vi "Simple_DAQ_AnalogIO.ProcCases.vi"(0 "i ref in":refnum<vi>, 1 "selector":string, 2 "Data":T1, 3 "call cluster":T2={"Object"="", "Selector"="", "CallType"=enum."synchronous", "Async Object"="", "Async Selector"="", "Data Descriptor"="", "Data"=[], "Error #"=0, "Expire"=0}, 5 "error in (no error)":errorcluster) -> (14 "i ref out":refnum<vi>, 17 "answer cluster":T2={"Object"="", "Selector"="", "CallType"=enum."synchronous", "Async Object"="", "Async Selector"="", "Data Descriptor"="", "Data"=[], "Error #"=0, "Expire"=0}, 19 "error out":errorcluster)   [LabVIEW 2014, in "Simple_DAQ_AnalogIO.lvlib"]
doc: "This method is called by a process from within the default case in the event loop. The methods of a class that are linked to events will be called from THIS method. Add your code here."
uses:
  Simple_DAQ_AnalogIO.lvlib
  CS_Core/CSSystem/CoreDefs/CoreDefs.call_type.ctl
  CS_Core/BaseProcess/BaseProcess.descriptor string definition.ctl
  CS_Core/CSSystem/CoreDefs/CoreDefs.rawDataType.ctl
  CS_Core/CSSystem/CoreLib/CoreLib.string 2 byte array.vi
  CS_Core/CSSystem/CoreLib/CoreLib.double 2 byte array.vi
  CS_Core/CSSystem/CoreLib/CoreLib.byte array 2 double.vi
  CS_Core/CSSystem/CoreLib/CoreLib.byte array 2 int.vi
  CS_Core/CSSystem/CoreLib/CoreLib.lvlib
  CS_Core/BaseProcess/BaseProcess.lvlib
  CS_Core/CSApplicationBaseClasses/PSChannelBase/PSChannelBase.lvlib
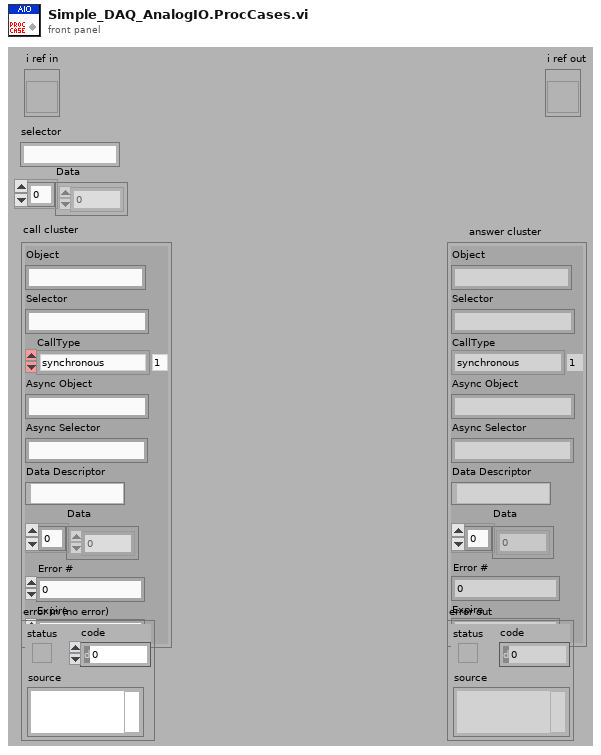
[diagram p1: front panel]
types:
  T1 = typedef "CoreDefs.rawDataType.ctl" = i8[]
  T2 = typedef "CoreDefs.call_type.ctl" = cluster{"Object":string, "Selector":string, "CallType":enum16{"simple", "synchronous", "asynchronous"}, "Async Object":string, "Async Selector":string, "Data Descriptor":T3, "Data":T1, "Error #":i32, "Expire":u32}
  T3 = typedef "BaseProcess.lvlib/BaseProcess.descriptor string definition.ctl" = string
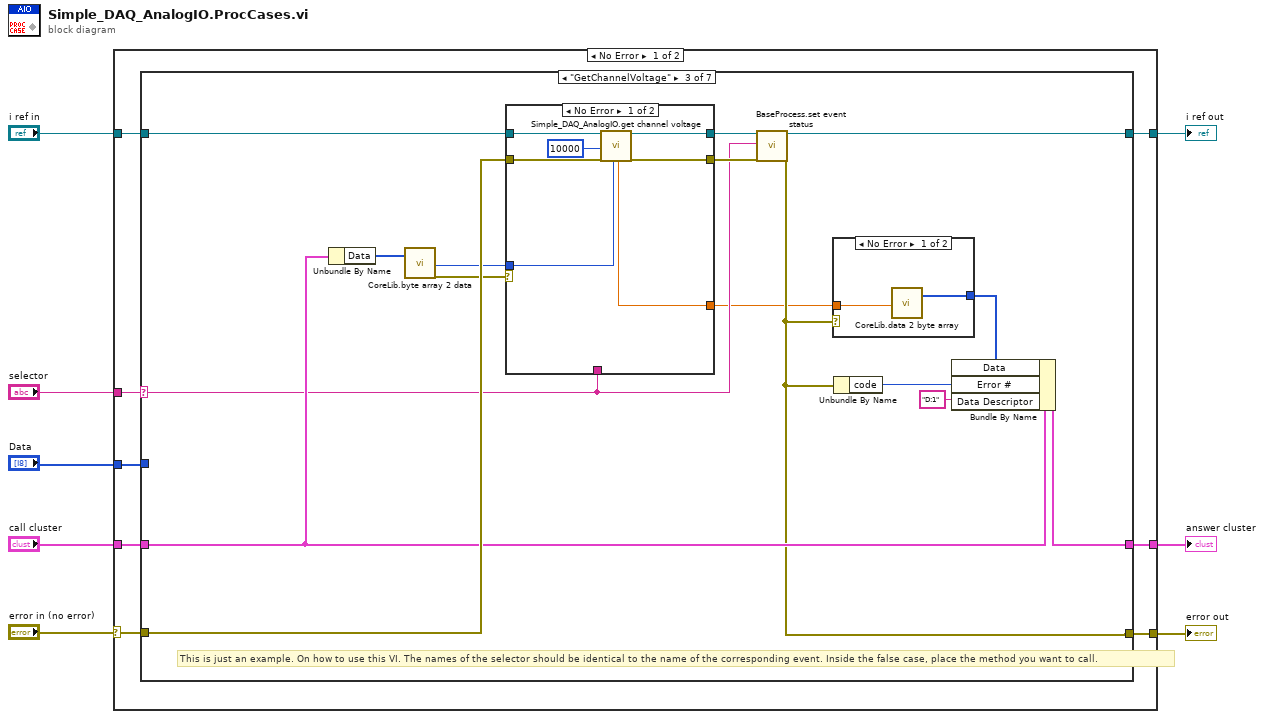
[diagram p0: block diagram]
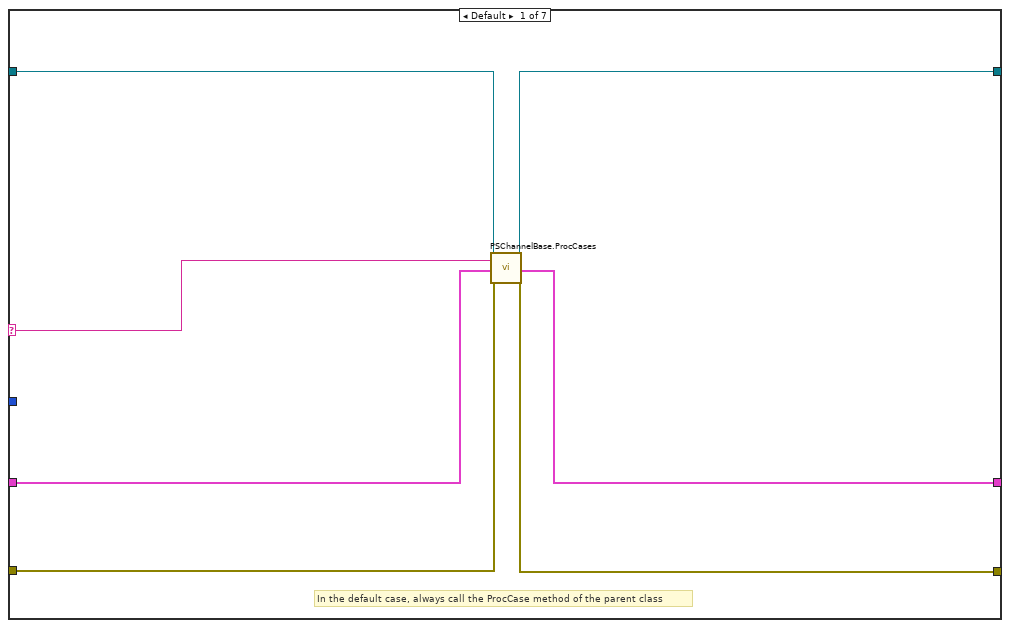
[diagram p2: hidden frame]
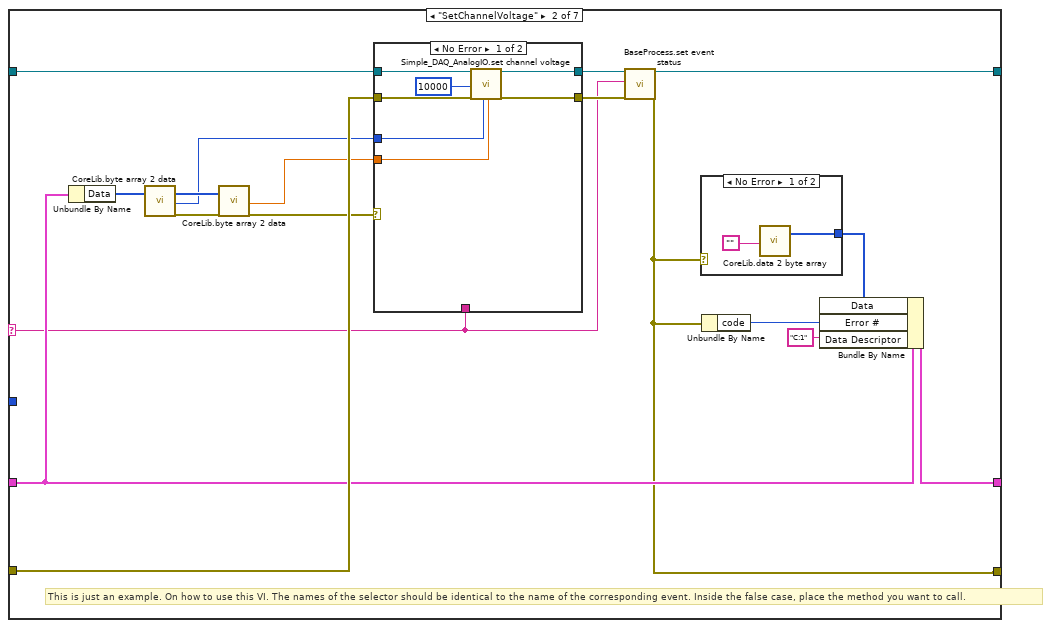
[diagram p3: hidden frame]
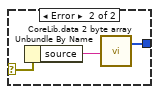
[diagram p4: hidden frame]
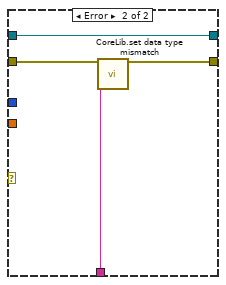
[diagram p5: hidden frame]
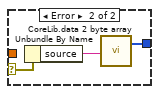
[diagram p6: hidden frame]
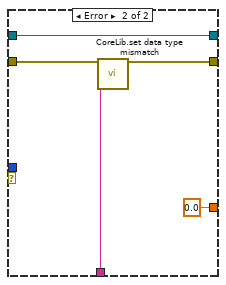
[diagram p7: hidden frame]
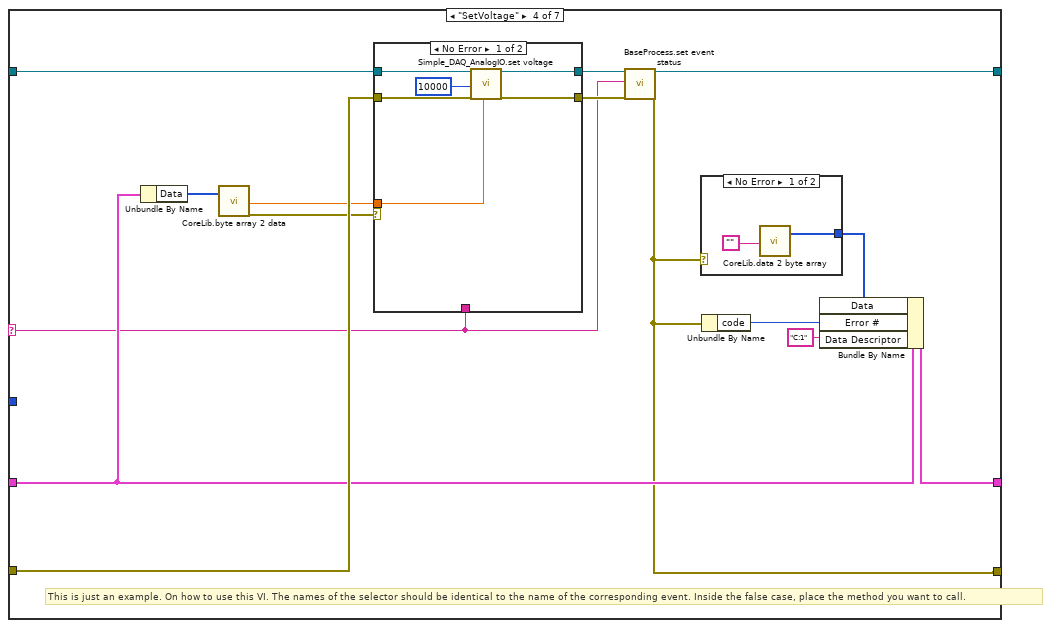
[diagram p8: hidden frame]
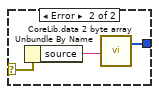
[diagram p9: hidden frame]
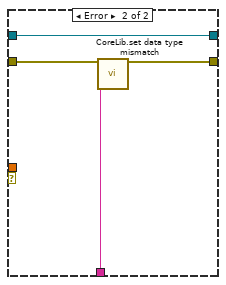
[diagram p10: hidden frame]
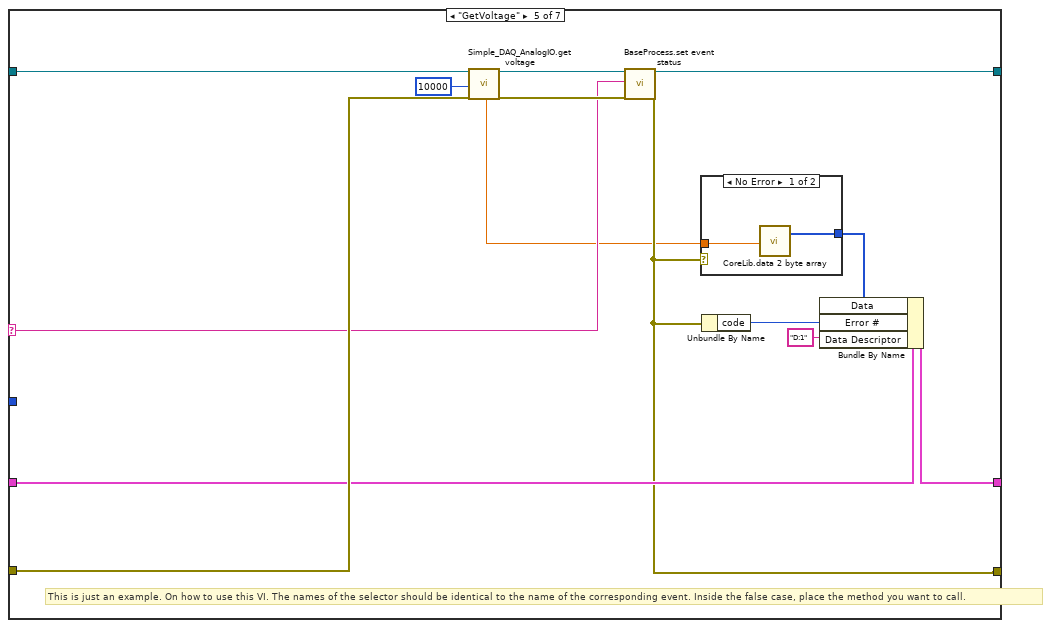
[diagram p11: hidden frame]
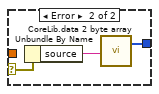
[diagram p12: hidden frame]
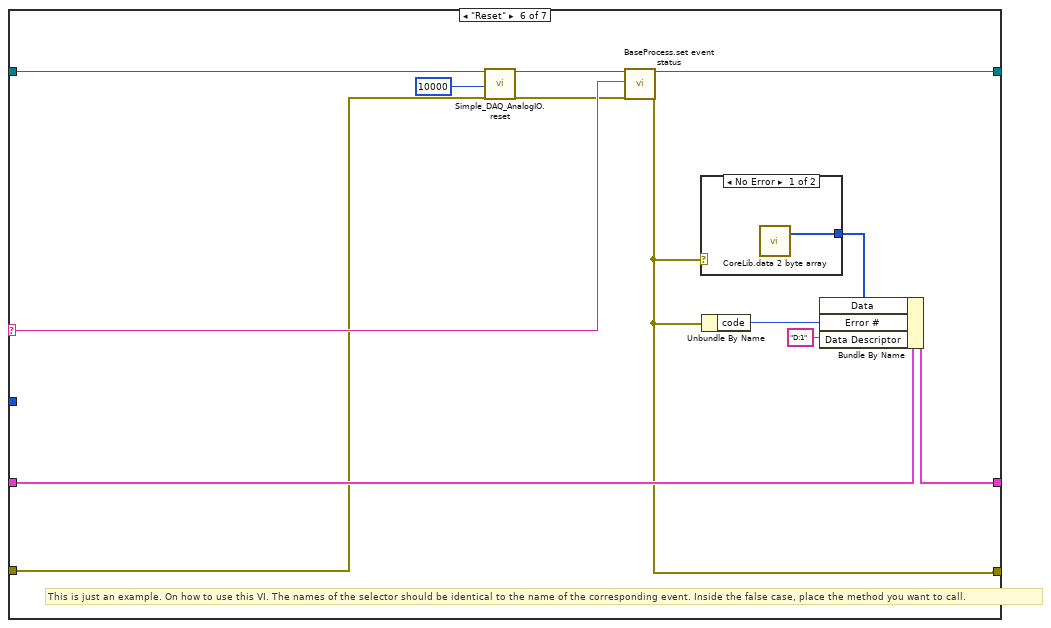
[diagram p13: hidden frame]
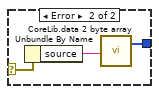
[diagram p14: hidden frame]
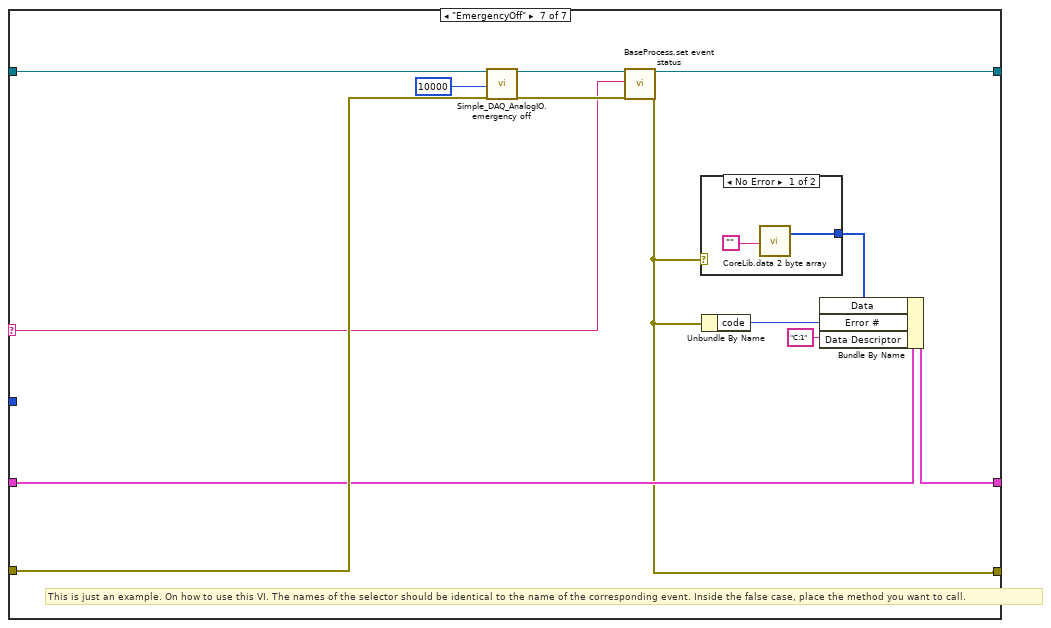
[diagram p15: hidden frame]
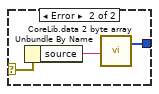
[diagram p16: hidden frame]
diagram:
  n1 = case shown="No Error" "error in (no error)" {
    selector: "error in (no error)" -> [w9 w175]
    tunnel: "selector" -> [w16 _]
    tunnel: [w15 w176] -> w7
    tunnel: "Data" -> [w14 _]
    tunnel: "call cluster" -> [w13 w176]
    tunnel: "i ref in" -> [w12 w177]
    tunnel: [w11 w177] -> w3
    tunnel: [w10 w175] -> w2
    frame No Error {
      n2 = case shown="\"GetChannelVoltage\"" w16 {
        selector: w16 -> [w18 w32 w64 w96 w125 w147 w160]
        tunnel: w14 -> [_ _ _ _ _ _ _]
        tunnel: w12 -> [w17 w41 w73 w105 w134 w144 w169]
        tunnel: [w23 w31 w63 w95 w124 w146 w159] -> w11
        tunnel: w13 -> [w19 w38 w70 w102 w131 w151 w166]
        tunnel: [w20 w37 w69 w101 w130 w150 w165] -> w15
        tunnel: w9 -> [w22 w40 w72 w104 w133 w141 w168]
        tunnel: [w21 w33 w65 w97 w126 w148 w161] -> w10
        frame Default {
          # "In the default case, always call the ProcCase method of the parent class"
          n3 = call "PSChannelBase.ProcCases.vi"("i ref in"=w17, "selector"=w18, "call cluster"=w19, "error in (no error)"=w22) -> ("i ref out"=w23:refnum<vi>, "answer cluster"=w20:T2, "error out"=w21:errorcluster)  [unwired: 13 in]
        }
        frame "SetChannelVoltage" {
          # "This is just an example. On how to use this VI. The names of the selector should be identical to the name of the corresponding event. Inside the false case, place the method you want to call."
          n4 = Unbundle By Name(w38) -> ("Data"=w29:T1)
          n5 = call-poly "CoreLib.byte array 2 data.vi"("byteArray"=w29) -> ("byteArray out"=w27:T1, "i32"=w25:i32, "error out"=w28:errorcluster)  [unwired: 16 in]
          n6 = call-poly "CoreLib.byte array 2 data.vi"("byteArray"=w27, "error in (no error)"=w28) -> ("d64"=w24:dbl, "error out"=w26:errorcluster)  [unwired: 15 in, 1 out]
          n7 = case shown="No Error" w26 {
            tunnel: [w51 w57] -> w35
            tunnel: w41 -> [w52 w57]
            tunnel: w40 -> [w53 w56]
            tunnel: [w50 w55] -> w34
            tunnel: w24 -> [w47 _]
            tunnel: w32 -> [_ w54]
            tunnel: w25 -> [w48 _]
            frame No Error {
              n8 = call "Simple_DAQ_AnalogIO.set channel voltage.vi"("i ref in"=w52, "Timeout"=10000, "error in"=w53, "channel_index"=w48, "voltage"=w47) -> ("i ref out"=w51:refnum<vi>, "error out"=w50:errorcluster)  [unwired: 12 in, 1 out]
            }
            frame Error {
              n9 = call "CoreLib.set data type mismatch.vi"("error in (no error)"=w56, "error source"=w54) -> ("error out"=w55:errorcluster)  [unwired: 17 in]
            }
          }
          n10 = call "BaseProcess.set event status.vi"("i ref in"=w35, "EventStatus"=w32, "error in (no error)"=w34) -> ("i ref out"=w31:refnum<vi>, "error out"=w33:errorcluster)  [unwired: 14 in, 1 out]
          n11 = case shown="No Error" w33 {
            selector: w33 -> [_ w46]
            tunnel: [w43 w45] -> w36
            frame No Error {
              n12 = call-poly "CoreLib.data 2 byte array.vi"("string"="") -> ("byteArray out"=w43:T1)  [unwired: 18 in]
            }
            frame Error {
              n13 = Unbundle By Name(w46) -> ("source"=w44:string)
              n14 = call-poly "CoreLib.data 2 byte array.vi"("string"=w44) -> ("byteArray out"=w45:T1)  [unwired: 18 in]
            }
          }
          n15 = Unbundle By Name(w33) -> ("code"=w39:i32)
          n16 = Bundle By Name(cluster=w38, "Data"=w36, "Error #"=w39, "Data Descriptor"="C:1") -> (w37:T2)
        }
        frame "GetChannelVoltage" {
          # "This is just an example. On how to use this VI. The names of the selector should be identical to the name of the corresponding event. Inside the false case, place the method you want to call."
          n17 = Unbundle By Name(w70) -> ("Data"=w61:T1)
          n18 = call-poly "CoreLib.byte array 2 data.vi"("byteArray"=w61) -> ("i32"=w60:i32, "error out"=w59:errorcluster)  [unwired: 16 in, 1 out]
          n19 = case shown="No Error" w59 {
            tunnel: [w83 w90] -> w67
            tunnel: w73 -> [w84 w90]
            tunnel: w72 -> [w85 w89]
            tunnel: [w82 w88] -> w66
            tunnel: w64 -> [_ w87]
            tunnel: w60 -> [w80 _]
            tunnel: [w79 0.0 ("voltage")] -> w58
            frame No Error {
              n20 = call "Simple_DAQ_AnalogIO.get channel voltage.vi"("i ref in"=w84, "Timeout"=10000, "error in"=w85, "channel_index"=w80) -> ("voltage"=w79:dbl, "i ref out"=w83:refnum<vi>, "error out"=w82:errorcluster)  [unwired: 12 in, 1 out]
            }
            frame Error {
              n21 = call "CoreLib.set data type mismatch.vi"("error in (no error)"=w89, "error source"=w87) -> ("error out"=w88:errorcluster)  [unwired: 17 in]
            }
          }
          n22 = call "BaseProcess.set event status.vi"("i ref in"=w67, "EventStatus"=w64, "error in (no error)"=w66) -> ("i ref out"=w63:refnum<vi>, "error out"=w65:errorcluster)  [unwired: 14 in, 1 out]
          n23 = case shown="No Error" w65 {
            selector: w65 -> [_ w78]
            tunnel: [w75 w77] -> w68
            tunnel: w58 -> [w74 _]
            frame No Error {
              n24 = call-poly "CoreLib.data 2 byte array.vi"("f64"=w74) -> ("byteArray out"=w75:T1)  [unwired: 18 in]
            }
            frame Error {
              n25 = Unbundle By Name(w78) -> ("source"=w76:string)
              n26 = call-poly "CoreLib.data 2 byte array.vi"("string"=w76) -> ("byteArray out"=w77:T1)  [unwired: 18 in]
            }
          }
          n27 = Unbundle By Name(w65) -> ("code"=w71:i32)
          n28 = Bundle By Name(cluster=w70, "Data"=w68, "Error #"=w71, "Data Descriptor"="D:1") -> (w69:T2)
        }
        frame "SetVoltage" {
          # "This is just an example. On how to use this VI. The names of the selector should be identical to the name of the corresponding event. Inside the false case, place the method you want to call."
          n29 = Unbundle By Name(w102) -> ("Data"=w91:T1)
          n30 = call-poly "CoreLib.byte array 2 data.vi"("byteArray"=w91) -> ("d64"=w92:dbl, "error out"=w93:errorcluster)  [unwired: 16 in, 1 out]
          n31 = case shown="No Error" w93 {
            tunnel: [w114 w120] -> w99
            tunnel: w105 -> [w115 w120]
            tunnel: w104 -> [w116 w119]
            tunnel: [w113 w118] -> w98
            tunnel: w92 -> [w111 _]
            tunnel: w96 -> [_ w117]
            frame No Error {
              n32 = call "Simple_DAQ_AnalogIO.set voltage.vi"("i ref in"=w115, "Timeout"=10000, "error in"=w116, "voltage"=w111) -> ("i ref out"=w114:refnum<vi>, "error out"=w113:errorcluster)  [unwired: 13 in, 1 out]
            }
            frame Error {
              n33 = call "CoreLib.set data type mismatch.vi"("error in (no error)"=w119, "error source"=w117) -> ("error out"=w118:errorcluster)  [unwired: 17 in]
            }
          }
          n34 = call "BaseProcess.set event status.vi"("i ref in"=w99, "EventStatus"=w96, "error in (no error)"=w98) -> ("i ref out"=w95:refnum<vi>, "error out"=w97:errorcluster)  [unwired: 14 in, 1 out]
          n35 = case shown="No Error" w97 {
            selector: w97 -> [_ w110]
            tunnel: [w107 w109] -> w100
            frame No Error {
              n36 = call-poly "CoreLib.data 2 byte array.vi"("string"="") -> ("byteArray out"=w107:T1)  [unwired: 18 in]
            }
            frame Error {
              n37 = Unbundle By Name(w110) -> ("source"=w108:string)
              n38 = call-poly "CoreLib.data 2 byte array.vi"("string"=w108) -> ("byteArray out"=w109:T1)  [unwired: 18 in]
            }
          }
          n39 = Unbundle By Name(w97) -> ("code"=w103:i32)
          n40 = Bundle By Name(cluster=w102, "Data"=w100, "Error #"=w103, "Data Descriptor"="C:1") -> (w101:T2)
        }
        frame "GetVoltage" {
          # "This is just an example. On how to use this VI. The names of the selector should be identical to the name of the corresponding event. Inside the false case, place the method you want to call."
          n41 = call "Simple_DAQ_AnalogIO.get voltage.vi"("i ref in"=w134, "Timeout"=10000, "error in"=w133) -> ("voltage"=w122:dbl, "i ref out"=w128:refnum<vi>, "error out"=w127:errorcluster)  [unwired: 13 in, 1 out]
          n42 = call "BaseProcess.set event status.vi"("i ref in"=w128, "EventStatus"=w125, "error in (no error)"=w127) -> ("i ref out"=w124:refnum<vi>, "error out"=w126:errorcluster)  [unwired: 14 in, 1 out]
          n43 = case shown="No Error" w126 {
            selector: w126 -> [_ w139]
            tunnel: [w136 w138] -> w129
            tunnel: w122 -> [w135 _]
            frame No Error {
              n44 = call-poly "CoreLib.data 2 byte array.vi"("f64"=w135) -> ("byteArray out"=w136:T1)  [unwired: 18 in]
            }
            frame Error {
              n45 = Unbundle By Name(w139) -> ("source"=w137:string)
              n46 = call-poly "CoreLib.data 2 byte array.vi"("string"=w137) -> ("byteArray out"=w138:T1)  [unwired: 18 in]
            }
          }
          n47 = Unbundle By Name(w126) -> ("code"=w132:i32)
          n48 = Bundle By Name(cluster=w131, "Data"=w129, "Error #"=w132, "Data Descriptor"="D:1") -> (w130:T2)
        }
        frame "Reset" {
          # "This is just an example. On how to use this VI. The names of the selector should be identical to the name of the corresponding event. Inside the false case, place the method you want to call."
          n49 = call "Simple_DAQ_AnalogIO.reset.vi"("i ref in"=w144, "Timeout"=10000, "error in"=w141) -> ("i ref out"=w143:refnum<vi>, "error out"=w142:errorcluster)  [unwired: 14 in, 1 out]
          n50 = call "BaseProcess.set event status.vi"("i ref in"=w143, "EventStatus"=w147, "error in (no error)"=w142) -> ("i ref out"=w146:refnum<vi>, "error out"=w148:errorcluster)  [unwired: 14 in, 1 out]
          n51 = case shown="No Error" w148 {
            selector: w148 -> [_ w156]
            tunnel: [w153 w155] -> w149
            frame No Error {
              n52 = call-poly "CoreLib.data 2 byte array.vi"() -> ("byteArray out"=w153:T1)  [unwired: 19 in]
            }
            frame Error {
              n53 = Unbundle By Name(w156) -> ("source"=w154:string)
              n54 = call-poly "CoreLib.data 2 byte array.vi"("string"=w154) -> ("byteArray out"=w155:T1)  [unwired: 18 in]
            }
          }
          n55 = Unbundle By Name(w148) -> ("code"=w152:i32)
          n56 = Bundle By Name(cluster=w151, "Data"=w149, "Error #"=w152, "Data Descriptor"="D:1") -> (w150:T2)
        }
        frame "EmergencyOff" {
          # "This is just an example. On how to use this VI. The names of the selector should be identical to the name of the corresponding event. Inside the false case, place the method you want to call."
          n57 = call "Simple_DAQ_AnalogIO.emergency off.vi"("i ref in"=w169, "Timeout"=10000, "error in"=w168) -> ("i ref out"=w163:refnum<vi>, "error out"=w162:errorcluster)  [unwired: 14 in, 1 out]
          n58 = call "BaseProcess.set event status.vi"("i ref in"=w163, "EventStatus"=w160, "error in (no error)"=w162) -> ("i ref out"=w159:refnum<vi>, "error out"=w161:errorcluster)  [unwired: 14 in, 1 out]
          n59 = case shown="No Error" w161 {
            selector: w161 -> [_ w174]
            tunnel: [w171 w173] -> w164
            frame No Error {
              n60 = call-poly "CoreLib.data 2 byte array.vi"("string"="") -> ("byteArray out"=w171:T1)  [unwired: 18 in]
            }
            frame Error {
              n61 = Unbundle By Name(w174) -> ("source"=w172:string)
              n62 = call-poly "CoreLib.data 2 byte array.vi"("string"=w172) -> ("byteArray out"=w173:T1)  [unwired: 18 in]
            }
          }
          n63 = Unbundle By Name(w161) -> ("code"=w167:i32)
          n64 = Bundle By Name(cluster=w166, "Data"=w164, "Error #"=w167, "Data Descriptor"="C:1") -> (w165:T2)
        }
      }
    }
    frame Error {
    }
  }
  "answer cluster" <- w7
  "i ref out" <- w3
  "error out" <- w2
